vi "DisplaySet.vi"(7 "参数查询(0)/设置(1)":bool, 8 "error in (no error)":errorcluster caption="错误输入（无错误）", 9 "设置参数":string, 10 "DISPLAY命令子系统":string(combo), 11 "VISA资源名称":refnum<visa-resource-name>) -> (0 "error out":errorcluster caption="错误输出", 1 "查询返回字节数":u32, 2 "查询返回":string, 3 "VISA资源名称 2":refnum<visa-resource-name>)   [LabVIEW 2018]
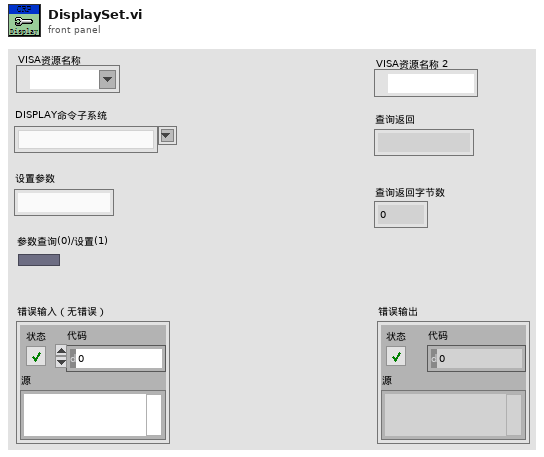
[diagram p1: front panel]
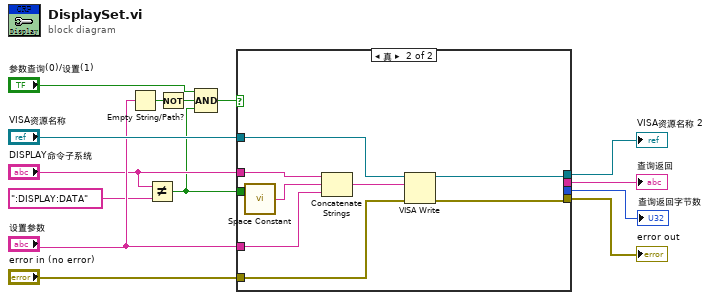
[diagram p0: block diagram]
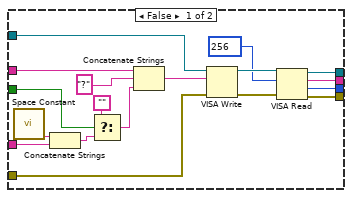
[diagram p2: hidden frame]
diagram:
  n1 = Empty String/Path?(string/path="设置参数") -> (empty?=w9:bool)
  n2 = Not Equal?(x="DISPLAY命令子系统", y=":DISPLAY:DATA" ("x")) -> (x != y?=w2:bool)
  n3 = Not(x=w9) -> (.not. x?=w1:bool)
  n4 = Compound Arithmetic op=AND ("复合运算")("参数查询(0)/设置(1)", w1, w2) -> (w8:bool)
  n5 = case shown="真" w8 {
    tunnel: "设置参数" -> [w18 w40]
    tunnel: "DISPLAY命令子系统" -> [w32 w38]
    tunnel: "VISA资源名称" -> [w29 w37]
    tunnel: "error in (no error)" -> [w28 w35]
    tunnel: [w24 w33] -> w10
    tunnel: [w23 w34] -> w11
    tunnel: [w22 _] -> w12
    tunnel: [w21 _] -> w6
    tunnel: w2 -> [w15 _]
    frame False {
      n6 = call <vilib>:"Space Constant.vi"() -> ("String"=w19:string)
      n7 = Concatenate Strings(w19, w18) -> (w17:string)
      n8 = Select(t="", s=w15, f=w17) -> (s? t:f=w20:string)
      n9 = Concatenate Strings(w32, "?" ("字符串"), w20) -> (w30:string)
      n10 = VISA Write(VISA resource name=w29, write buffer=w30, error in (no error)=w28) -> (VISA resource name out=w27:refnum<visa-resource-name>, error out=w26:errorcluster)  [unwired: 1 out]
      n11 = VISA Read(VISA resource name=w27, byte count=u32 256 ("字节总数"), error in (no error)=w26) -> (VISA resource name out=w23:refnum<visa-resource-name>, read buffer=w22:string, return count=w21:u32, error out=w24:errorcluster)
    }
    frame True {
      n12 = call <vilib>:"Space Constant.vi"() -> ("String"=w39:string)
      n13 = Concatenate Strings(w38, w39, w40) -> (w36:string)
      n14 = VISA Write(VISA resource name=w37, write buffer=w36, error in (no error)=w35) -> (VISA resource name out=w34:refnum<visa-resource-name>, error out=w33:errorcluster)  [unwired: 1 out]
    }
  }
  "VISA资源名称 2" <- w11
  "error out" <- w10
  "查询返回" <- w12
  "查询返回字节数" <- w6
